vi "Exit.vi"(8 "error in (no error)":errorcluster, 10 "Context in":refnum<class "Context.lvclass">, 11 "Logging in":refnum<class "Logging.lvclass">) -> (0 "error out":errorcluster, 2 "Context out":refnum<class "Context.lvclass">, 3 "Logging out":refnum<class "Logging.lvclass">)   [LabVIEW 2024, in "State.lvlib" / "Logging.lvclass"]
uses:
  Logging.lvclass
  Context/Context/Context.lvclass
  Logging.lvclass/Logging.ctl
panel:
  # "LOGGING EXIT"
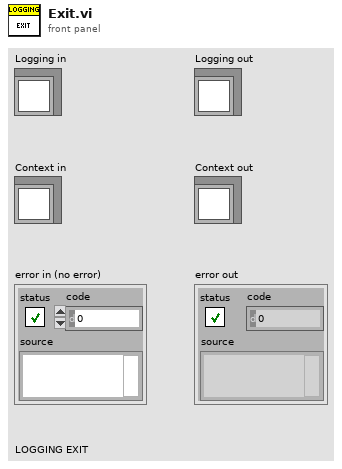
[diagram p1: front panel]
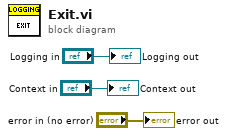
[diagram p0: block diagram]
diagram:
  "error out" <- "error in (no error)"
  "Logging out" <- "Logging in"
  "Context out" <- "Context in"
